vi "ReadBase.vi"(8 "error in (no error)":errorcluster, 10 "Request Number of Message":i32, 11 "Konvolucio MCAN120803 Adapter Class in":refnum<class "Konvolucio MCAN120803 Adapter Class.lvclass">) -> (0 "error out":errorcluster, 2 "Messages":T1[](array[typedef]) {"Data" format="%02x"; "Arbitration Id" format="%03x"}, 3 "Konvolucio MCAN120803 Adapter Class out":refnum<class "Konvolucio MCAN120803 Adapter Class.lvclass">)   [LabVIEW 2011, in "Konvolucio MCAN120803 Adapter Class.lvclass"]
uses:
  Konvolucio MCAN120803 Adapter Class.lvclass
  National Instruments USB-8473 Adapter/MessageType.ctl
  Generic CAN Adapter/GenericCanAdapterClass.lvclass
  Konvolucio MCAN120803 Adapter Class.lvclass/Konvolucio MCAN120803 Adapter Class.ctl
  <instrlib>/Konvolucio MCAN120803/Konvolucio MCAN120803.lvlib
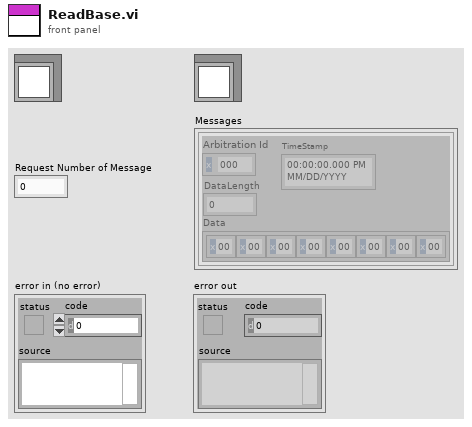
[diagram p1: front panel]
types:
  T1 = typedef "GenericCanAdapterClass.lvclass/MessageType.ctl" = cluster{"Arbitration Id":u32, "Data":u8[], "DataLength":u16, "TimeStamp":timestamp}
  T2 = typedef "Konvolucio MCAN120803.lvlib/MessageType.ctl" = cluster{"TimeStamp":timestamp, "ArbitrationId":u32, "IsRemote":u8, "DataLength":u8, "Data":u8[]}
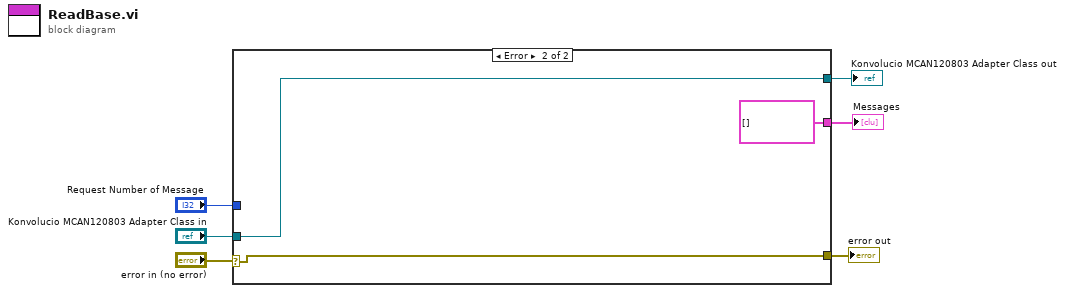
[diagram p0: block diagram]
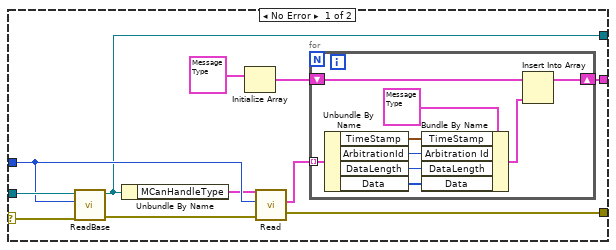
[diagram p2: hidden frame]
diagram:
  n1 = case shown="Error" "error in (no error)" {
    selector: "error in (no error)" -> [w7 w28]
    tunnel: "Konvolucio MCAN120803 Adapter Class in" -> [w17 w29]
    tunnel: "Request Number of Message" -> [w15 _]
    tunnel: [w14 w29] -> w4
    tunnel: [w12 w28] -> w3
    tunnel: [w8 T1[] []] -> w2
    frame No Error {
      n2 = call-parent "ReadBase.vi"("error in (no error)"=w7, "Request Number of Message"=w15, "GenericCanAdapterClass in"=w17) -> ("error out"=w16:errorcluster, "GenericCanAdapterClass out"=w14:refnum<class "Konvolucio MCAN120803 Adapter Class.lvclass">)  [unwired: 6 in, 1 out]
      n3 = Unbundle By Name(w14) -> ("MCanHandleType"=w13:cluster{"MCanAdapter":refnum<k24>})
      n4 = Initialize Array(T1 {"Arbitration Id"=0, "Data"=[0, 0, 0, 0, 0, 0, 0, 0], "DataLength"=0, "TimeStamp"=timestamp(0 s since 1904-01-01)} ("MessageType")) -> (w9:T1[])  [unwired: 1 in]
      n5 = call <instrlib>:"Read.vi"("error in"=w16, "Request Number of Message"=w15, "CanHandleIn"=w13) -> ("error out"=w12:errorcluster, "Messages"=w11:T2[])  [unwired: 6 in, 1 out]
      n6 = for {
        tunnel: w11 -> [w24] mode=indexing
        shift-right: [w25] -> w8
        shift-left: w9 -> [w26]
        n7 = Unbundle By Name(w24) -> ("TimeStamp"=w22:timestamp, "ArbitrationId"=w21:u32, "DataLength"=w20:u8, "Data"=w19:u8[])
        n8 = Bundle By Name(cluster=T1 {"Arbitration Id"=0, "Data"=[0, 0, 0, 0, 0, 0, 0, 0], "DataLength"=0, "TimeStamp"=timestamp(0 s since 1904-01-01)} ("MessageType"), "TimeStamp"=w22, "Arbitration Id"=w21, "DataLength"=w20, "Data"=w19) -> (w18:T1)
        n9 = Insert Into Array(array=w26, new element=w18) -> (w25:T1[])  [unwired: 1 in]
      }
    }
    frame Error {
    }
  }
  "error out" <- w3
  "Konvolucio MCAN120803 Adapter Class out" <- w4
  "Messages" <- w2
